vi "UHR-Fleezers Control (host) - 10.5.vi"() -> ()   [LabVIEW 2011] (continued)
                          n1375 = local read "BD 2 Frequency 3 (MHz)"() -> (w2101:dbl)
                          n1376 = local write "Trap Delta (MHz)"(w2098) -> ()
                          n1377 = call "set RF board frequency - interlace.vi"("Board 2 Frequency Limits"=w2099, "Board 1 Frequency Limits"=w2100, "FPGA VI Reference In"=w2107, "Board 2 Frequency 3 (MHz)"=w2101, "Board 1 Frequency 3 (MHz)"=w2106, "Board 2 Frequency 2 (MHz)"=w2102, "Board 2 Frequency 1 (MHz)"=w2103, "Board 1 Frequency 2 (MHz)"=w2104, "Board 1 Frequency 1  (MHz)"=w2105) -> ()  [unwired: 1 in, 2 out]
                          n1378 = local write "BD 2 Frequency 1 (MHz)"(w2103) -> ()
                          n1379 = local write "BD 1 Frequency 1 (MHz)"(w2105) -> ()
                        }
                      }
                    }
                    frame True {
                    }
                  }
                }
                event Mouse Up {
                  n1380 = event-data() -> ("Button"=w2108:u16)  [unwired: 8 out]
                  n1381 = case shown="3" w2108 {
                    tunnel: [FALSE TRUE] -> w2109
                    frame 0, Default {
                    }
                    frame 3 {
                      n1382 = local read "Trap Delta (MHz)"() -> (w2111:dbl)
                      n1383 = property on="Initial delta (MHz)" class="DigNum (strict)"("Val(Sgnl)"=w2111) -> ()  [unwired: 2 in, 2 out]
                      n1384 = local write "Manipulating Trap"(FALSE ("Manipulating Trap")) -> ()
                    }
                  }
                }
              }
            }
          }
        }
      }
      event Mouse Move {
        n1385 = event-data() -> ()  [unwired: 6 out]
      }
    }
    n1386 = local read "Stop All"() -> (w1930:bool)
    n1387 = node-c288() -> ()  [unwired: 2 out]
  }
  n1388 = timed-loop "Oscillate Trap/AOM (fishing, debugging)" {
    tunnel: w40 -> [w2115]
    tunnel: [w2114] -> w85
    timing: w80 -> [_]
    timing-out: [_] -> w79
    stop <- w2114 stop-if-true
    n1389 = node-c288() -> ()  [unwired: 2 out]
    n1390 = event shown="[0] \"Oscillate Set 1\", \"Fish for Tether\": Value Change" {
      selector: _ -> [_ _ _]
      dyn-events: _ -> [_ _ _]
      timeout: _ -> [_ _ _]
      tunnel: w2115 -> [w2122 _ _]
      tunnel: [FALSE ("Stop All") _ w2411] -> w2114
      event "Oscillate Set 1", "Fish for Tether": Value Change {
        n1391 = event-data() -> ()  [unwired: 6 out]
        n1392 = local read "Oscillate Set 1"() -> (w2121:bool)
        n1393 = Or(x=w2121, y="Fish for Tether") -> (x .or. y?=w2119:bool)
        n1394 = case shown="True" w2119 {
          tunnel: w2122 -> [_ w2125]
          tunnel: "Fish for Tether" -> [_ w2124]
          frame False {
          }
          frame True {
            n1395 = case shown="True" w2124 {
              selector: w2124 -> [w2128 w2135]
              tunnel: [w2128 w2135] -> w2123
              frame False {
              }
              frame True {
                n1396 = local write "Scan axis 2"(TRUE) -> ()
                n1397 = local write "Tether"(FALSE ("Tether")) -> ()
                n1398 = property on="Trap Delta (MHz)" class="DigNum (strict)"("Val(Sgnl)"="Furthest Delta (MHz)") -> ()  [unwired: 2 in, 2 out]
                n1399 = local read "Sample Channel\nFlow"() -> (w2132:bool)
                n1400 = Not(x=w2132) -> (.not. x?=w2130:bool)
                n1401 = And(x=w2130, y="Flow ON during \nfishing?") -> (x .and. y?=w2129:bool)
                n1402 = Wait (ms)(milliseconds to wait=u32 500) -> ()  [unwired: 1 out]
                n1403 = case shown="True" w2129 {
                  selector: w2129 -> [_ w2138]
                  frame False {
                  }
                  frame True {
                    n1404 = property on="Sample Channel\nFlow" class="Bool (strict)"("Val(Sgnl)"=w2138) -> ()  [unwired: 2 in, 2 out]
                  }
                }
              }
            }
            n1405 = node-c288() -> (w2127:T21)  [unwired: 4 out]
            n1406 = timed-loop "Oscillate AOD" {
              timing: w2127 -> [_]
              timing-out: [_] -> w2126
              tunnel: w2125 -> [w2146]
              tunnel: w2123 -> [w2139]
              i -> [w2148]
              stop <- w2145 stop-if-true
              n1407 = node-c288() -> (w2147:i64)  [unwired: 1 out]
              n1408 = flat-sequence {
                tunnel: w2148 -> [w2175]
                tunnel: w2147 -> [w2174]
                tunnel: w2146 -> [w2153]
                tunnel: w2139 -> [w2156]
                tunnel: [w2156] -> w2144
                tunnel: [w2155] -> w2143
                tunnel: [w2152] -> w2142
                tunnel: [w2149] -> w2140
                tunnel: w2144 -> [w2211]
                tunnel: w2143 -> [w2209]
                tunnel: w2142 -> [w2208]
                tunnel: [w2207] -> w2141
                tunnel: w2140 -> [w2206]
                tunnel: [w2285] -> w2145
                tunnel: w2141 -> [w2284]
                frame #0 {
                  n1409 = Divide(x=w2174, y=i64 1000) -> (x/y=w2169:dbl)
                  n1410 = Multiply(x=w2169, y=w2175) -> (x*y=w2171:dbl)
                  n1411 = local read "BD 1 Frequency 2 (MHz)"() -> (w2154:dbl)
                  n1412 = Multiply(x="Osc. freq. (Hz)", y=6.283185307179586) -> (x*y=w2172:dbl)
                  n1413 = Multiply(x=w2172, y=w2171) -> (x*y=w2151:dbl)
                  n1414 = local read "BD 1 Frequency 1 (MHz)"() -> (w2159:dbl)
                  n1415 = case shown="True" w2156 {
                    tunnel: w2151 -> [w2181 w2186]
                    tunnel: w2159 -> [_ w2197]
                    tunnel: w2154 -> [_ w2198]
                    tunnel: [w2178 w2192] -> w2157
                    tunnel: [FALSE w2189] -> w2152
                    tunnel: [0.0 w2182] -> w2149
                    frame False {
                      n1416 = Sine(x=w2181) -> (sin(x)=w2179:dbl)
                      n1417 = Multiply(x=w2179, y="Osc. amp. (MHz)") -> (x*y=w2178:dbl)
                    }
                    frame True {
                      n1418 = Cosine(x=w2186) -> (cos(x)=w2201:dbl)
                      n1419 = Subtract(x=w2198, y=w2197) -> (x-y=w2196:dbl)
                      n1420 = Decrement(x=w2201) -> (x-1=w2200:dbl)
                      n1421 = Subtract(x=w2196, y="Closest Delta (MHz)") -> (x-y=w2193:dbl)
                      n1422 = Divide(x=w2200, y=-2.0) -> (x/y=w2194:dbl)
                      n1423 = Multiply(x=w2194, y=w2193) -> (x*y=w2192:dbl)
                      n1424 = local read "Vec Mean of T1 T2"() -> (w2188:dbl[])
                      n1425 = Greater?(x=w2188, y="Stop F (pN)") -> (0:w2190:bool[])
                      n1426 = Or Array Elements(Boolean array=w2190) -> (logical OR=w2189:bool)
                      n1427 = Divide(x=w2186, y=6.283185307179586) -> (x/y=w2185:dbl)
                      n1428 = Round Toward +Infinity(x=w2185) -> (ceil(x): smallest int >= x=w2182:dbl)
                      "Attempts" <- w2182
                      n1429 = Greater?(x=w2182, y="Attempt Limit") -> (0:w2184:bool)
                      n1430 = case shown="True" w2184 {
                        frame False {
                        }
                        frame True {
                          n1431 = local write "Fish for Tether"(FALSE ("Fish for Tether")) -> ()
                          n1432 = call <vilib>:"Beep.vi"() -> ()  [unwired: 3 in, 9 out]
                          n1433 = local read "Messages"() -> (w2203:string)
                          n1434 = call "Update messages.vi"("Message to add"="Tether fishing timeout." ("Messages"), "Old message string"=w2203) -> ("New message string"=→"Messages":string)
                        }
                      }
                    }
                  }
                  n1435 = local read "BD 2 Frequency 1 (MHz)"() -> (w2158:dbl)
                  n1436 = Select(t=w2159, s="Scan axis 2", f=w2158) -> (s? t:f=w2162:dbl)
                  n1437 = Add(x=w2157, y=w2162) -> (x+y=w2155:dbl)
                  n1438 = Select(t=w2155, s="Scan axis 2", f=w2159) -> (s? t:f=w2165:dbl)
                  n1439 = Select(t=w2158, s="Scan axis 2", f=w2155) -> (s? t:f=w2164:dbl)
                  n1440 = local read "Y RF Frequency Limits (MHz)"() -> (w2160:T16)
                  n1441 = local read "X RF Frequency Limits (MHz)"() -> (w2161:T16)
                  n1442 = local read "BD 1 Frequency 3 (MHz)"() -> (w2168:dbl)
                  n1443 = local read "BD 2 Frequency 2 (MHz)"() -> (w2167:dbl)
                  n1444 = local read "BD 2 Frequency 3 (MHz)"() -> (w2166:dbl)
                  n1445 = call "set RF board frequency - interlace.vi"("Board 2 Frequency Limits"=w2160, "Board 1 Frequency Limits"=w2161, "FPGA VI Reference In"=w2153, "Board 2 Frequency 3 (MHz)"=w2166, "Board 1 Frequency 3 (MHz)"=w2168, "Board 2 Frequency 2 (MHz)"=w2167, "Board 2 Frequency 1 (MHz)"=w2164, "Board 1 Frequency 2 (MHz)"=w2154, "Board 1 Frequency 1  (MHz)"=w2165) -> ()  [unwired: 1 in, 2 out]
                }
                frame #1 {
                  n1446 = And(x=w2211, y=w2208) -> (x .and. y?=w2210:bool)
                  n1447 = case "Only if were fishing and now formed tether" shown="True" w2210 {
                    tunnel: w2209 -> [w2213 w2230]
                    tunnel: [w2212 w2229] -> w2207
                    tunnel: w2206 -> [_ w2225]
                    frame False {
                      n1448 = local read "Fish for Tether"() -> (w2212:bool)
                      n1449 = case shown="False" w2212 {
                        tunnel: w2213 -> [w2214 _]
                        frame False {
                          n1450 = property on="BD 1 Frequency 1 (MHz)" class="DigNum (strict)"("Val(Sgnl)"=w2214) -> ()  [unwired: 2 in, 2 out]
                        }
                        frame True {
                        }
                      }
                    }
                    frame True {
                      w2229 = FALSE ("Fish for Tether")
                      n1451 = call <vilib>:"Beep.vi"() -> ()  [unwired: 3 in, 9 out]
                      n1452 = Number To Decimal String(number=w2225, width (-)=i16 1) -> (decimal integer string=w2223:string)
                      n1453 = Concatenate Strings("Formed tether in ", w2223, " attempt(s)." ("string")) -> (w2220:string)
                      n1454 = local read "Messages"() -> (w2227:string)
                      n1455 = local write "Fish for Tether"(w2229) -> ()
                      n1456 = call "Update messages.vi"("Message to add"=w2220, "Old message string"=w2227) -> ("New message string"=w2226:string)
                      n1457 = local write "Messages"(w2226) -> ()
                      n1458 = Get Date/Time In Seconds() -> (seconds since 1Jan1904=→"Time tether formed":timestamp)
                      n1459 = local read "Sample Channel\nFlow"() -> (w2218:bool)
                      n1460 = local read "Flow ON during \nfishing?"() -> (w2217:bool)
                      n1461 = And(x=w2218, y=w2217) -> (x .and. y?=w2216:bool)
                      n1462 = case shown="True" w2216 {
                        tunnel: [_ w2232] -> w2215
                        frame False {
                        }
                        frame True {
                          n1463 = property on="Sample Channel\nFlow" class="Bool (strict)"("Val(Sgnl)"=FALSE ("Value (Signaling)")) -> (error out=w2232:errorcluster)  [unwired: 2 in, 1 out]
                        }
                      }
                      n1464 = case shown="\"2\", \"3\", \"4\", \"5\", \"6\"" "Then..." {
                        selector: "Then..." -> [_ w2235]
                        tunnel: w2230 -> [w2234 _]
                        tunnel: w2215 -> [_ _]
                        frame "1", Default {
                          n1465 = property on="BD 1 Frequency 1 (MHz)" class="DigNum (strict)"("Val(Sgnl)"=w2234) -> ()  [unwired: 2 in, 2 out]
                        }
                        frame "2", "3", "4", "5", "6" {
                          n1466 = flat-sequence {
                            tunnel: w2235 -> [w2237]
                            frame #0 {
                              n1467 = property on="Trap Delta (MHz)" class="DigNum (strict)"("Val(Sgnl)"="Move to Delta 1 (MHz)") -> ()  [unwired: 2 in, 2 out]
                            }
                            frame #1 {
                              n1468 = case shown="\"5\", \"6\"" w2237 {
                                selector: w2237 -> [w2240 w2250 _]
                                frame "3", "4" {
                                n1469 = flat-sequence {
                                tunnel: w2240 -> [w2241]
                                tunnel: [w2241] -> w2238
                                tunnel: [w2243] -> w2239
                                tunnel: w2238 -> [w2243]
                                tunnel: w2239 -> [w2247]
                                frame #0 {
                                n1470 = property on="Green Laser ON/Interlacing" class="Bool (strict)"("Val(Sgnl)"=TRUE ("Value (Signaling)")) -> ()  [unwired: 2 in, 2 out]
                                }
                                frame #1 {
                                n1471 = Multiply(x="Wait Before Save (s)", y=u32 1000 ("x")) -> (x*y=w2245:u32)
                                n1472 = Wait (ms)(milliseconds to wait=w2245) -> ()  [unwired: 1 out]
                                }
                                frame #2 {
                                n1473 = property on="Start Saving" class="Bool (strict)"("Value"=TRUE ("Start Saving")) -> ()  [unwired: 2 in, 2 out]
                                n1474 = case shown="\"4\"" w2247 {
                                frame Default {
                                }
                                frame "4" {
                                n1475 = property on="Fl. Triggered..." class="Bool (strict)"("Val(Sgnl)"=TRUE ("Value (Signaling)")) -> ()  [unwired: 2 in, 2 out]
                                }
                                }
                                }
                                }
                                }
                                frame "5", "6" {
                                n1476 = stacked-sequence {
                                tunnel: w2250 -> [_ _ _ _ _ _ w2262]
                                frame #0 {
                                n1477 = Replace Array Subset(array=u32[] [0] ("Index Values"), new element="Raster Set Upon Tether", index=0) -> (w2251:u32[])
                                n1478 = property on="Saved AOD Raster Scan Parameter Sets" class="Arr (strict)"("Index Values"=w2251) -> ()  [unwired: 2 in, 2 out]
                                }
                                frame #1 {
                                n1479 = Wait (ms)(milliseconds to wait=u32 500) -> ()  [unwired: 1 out]
                                }
                                frame #2 {
                                n1480 = property on="Load parameters" class="Bool (strict)"("Val(Sgnl)"=TRUE ("Value (Signaling)")) -> ()  [unwired: 2 in, 2 out]
                                n1481 = case shown="True" "Green ON During Raster" {
                                frame False {
                                }
                                frame True {
                                n1482 = property on="Green Laser ON/Interlacing" class="Bool (strict)"("Val(Sgnl)"=TRUE ("Value (Signaling)")) -> ()  [unwired: 2 in, 2 out]
                                }
                                }
                                }
                                frame #3 {
                                n1483 = Wait (ms)(milliseconds to wait=u32 500) -> ()  [unwired: 1 out]
                                }
                                frame #4 {
                                n1484 = property on="Trap Raster Scan" class="Bool (strict)"("Val(Sgnl)"=TRUE ("Value (Signaling)")) -> ()  [unwired: 2 in, 2 out]
                                }
                                frame #5 {
                                n1485 = Wait (ms)(milliseconds to wait=u32 2000) -> ()  [unwired: 1 out]
                                }
                                frame #6 {
                                n1486 = flat-sequence {
                                tunnel: w2262 -> [w2269]
                                frame #0 {
                                n1487 = while {
                                stop <- w2265 stop-if-true
                                n1488 = local read "Raster Scanning..."() -> (w2264:bool)
                                n1489 = local read "Saving..."() -> (w2267:bool)
                                n1490 = Wait (ms)(milliseconds to wait=u32 100) -> ()  [unwired: 1 out]
                                n1491 = Not(x=w2267) -> (.not. x?=w2266:bool)
                                n1492 = Not(x=w2264) -> (.not. x?=w2263:bool)
                                n1493 = And(x=w2266, y=w2263) -> (x .and. y?=w2265:bool)
                                }
                                }
                                frame #1 {
                                n1494 = local read "Tether"() -> (w2270:bool)
                                n1495 = case shown="False" w2270 {
                                tunnel: w2269 -> [_ w2272]
                                frame False {
                                n1496 = property on="Fish for Tether" class="Bool (strict)"("Val(Sgnl)"="Fish again after \nraster break?") -> ()  [unwired: 2 in, 2 out]
                                }
                                frame True {
                                n1497 = stacked-sequence {
                                tunnel: w2272 -> [_ w2274 _ _]
                                frame #0 {
                                n1498 = property on="Trap Delta (MHz)" class="DigNum (strict)"("Val(Sgnl)"="Move to Delta 2 (MHz)") -> ()  [unwired: 2 in, 2 out]
                                }
                                frame #1 {
                                n1499 = flat-sequence {
                                tunnel: w2274 -> [w2276]
                                frame #0 {
                                n1500 = Wait (ms)(milliseconds to wait=u32 500) -> ()  [unwired: 1 out]
                                }
                                frame #1 {
                                n1501 = case shown="\"6\"" w2276 {
                                frame Default {
                                }
                                frame "6" {
                                n1502 = property on="Green Laser ON/Interlacing" class="Bool (strict)"("Val(Sgnl)"=TRUE ("Green Laser ON/Interlacing")) -> ()  [unwired: 2 in, 2 out]
                                }
                                }
                                }
                                frame #2 {
                                n1503 = Wait (ms)(milliseconds to wait=u32 500) -> ()  [unwired: 1 out]
                                }
                                frame #3 {
                                n1504 = local write "Start Saving"("Save at end (5, 6)") -> ()
                                }
                                }
                                }
                                frame #2 {
                                n1505 = local read "Bead Sep. Int. Time (s)"() -> (w2282:dbl)
                                n1506 = Multiply(x=w2282, y=1000.0) -> (x*y=w2281:dbl)
                                n1507 = Wait (ms)(milliseconds to wait=w2281) -> ()  [unwired: 1 out]
                                }
                                frame #3 {
                                n1508 = property on="Remove Offset" class="Bool (strict)"("Val(Sgnl)"=TRUE ("Value (Signaling)")) -> ()  [unwired: 2 in, 2 out]
                                }
                                }
                                }
                                }
                                }
                                }
                                }
                                }
                                }
                                frame "2", Default {
                                }
                              }
                            }
                          }
                        }
                      }
                      "Tether" <- "Tether Alarm?"
                    }
                  }
                }
                frame #2 {
                  n1509 = local read "Oscillate Set 1"() -> (w2289:bool)
                  n1510 = local read "Stop All"() -> (w2287:bool)
                  n1511 = Or(x=w2289, y=w2284) -> (x .or. y?=w2286:bool)
                  n1512 = Not(x=w2286) -> (.not. x?=w2288:bool)
                  n1513 = Compound Arithmetic op=OR(w2287, w2288) -> (w2285:bool)
                }
              }
              n1514 = node-c288() -> ()  [unwired: 2 out]
            }
            n1515 = node-c288(w2126) -> ()  [unwired: 1 out]
          }
        }
      }
      event "Fl. Triggered...": Value Change {
        n1516 = event-data() -> ()  [unwired: 7 out]
        n1517 = case shown="True" "Fl. Triggered..." {
          frame False {
          }
          frame True {
            n1518 = node-c288() -> (w2299:T21)  [unwired: 4 out]
            n1519 = timed-loop {
              timing: w2299 -> [_]
              timing-out: [_] -> w2298
              tunnel: "Action" -> [w2303]
              shift-right: [w2300] -> _
              shift-left: u8 255 -> [w2302]
              stop <- w2304 stop-if-true
              n1520 = node-c288() -> ()  [unwired: 2 out]
              n1521 = flat-sequence {
                tunnel: w2303 -> [w2316]
                tunnel: w2302 -> [w2313]
                tunnel: [w2312] -> w2301
                tunnel: [w2402] -> w2304
                tunnel: w2301 -> [w2401]
                tunnel: [w2401] -> w2300
                frame #0 {
                  n1522 = local read "Delta Fl. 2"() -> (w2307:dbl)
                  n1523 = local read "Delta Fl. 1"() -> (w2308:dbl)
                  n1524 = Select(t=w2308, s="APD to Watch", f=w2307) -> (s? t:f=w2306:dbl)
                  n1525 = Multiply(x="Fl. Delta Thresh. (kHz)", y=1000.0) -> (x*y=w2315:dbl)
                  n1526 = Greater?(x=w2306, y=w2315) -> (0:w2310:bool)
                  n1527 = Or(x="Force Yank", y=w2310) -> (x .or. y?=w2311:bool)
                  n1528 = case shown="True" w2311 {
                    tunnel: w2316 -> [_ w2326]
                    tunnel: w2313 -> [w2318 w2322]
                    tunnel: [w2318 w2319] -> w2312
                    frame False {
                    }
                    frame True {
                      n1529 = flat-sequence {
                        tunnel: w2323 -> [w2332]
                        tunnel: [w2332] -> w2327
                        tunnel: w2326 -> [w2331]
                        tunnel: [w2331] -> w2325
                        tunnel: [w2330] -> w2324
                        tunnel: w2322 -> [w2329]
                        tunnel: [w2328] -> w2321
                        tunnel: w2327 -> [w2357]
                        tunnel: w2325 -> [w2356]
                        tunnel: w2324 -> [w2355]
                        tunnel: w2321 -> [w2354]
                        tunnel: [w2354] -> w2320
                        tunnel: w2320 -> [w2399]
                        tunnel: [w2399] -> w2319
                        frame #0 {
                          n1530 = call <vilib>:"Beep.vi"() -> ()  [unwired: 3 in, 9 out]
                          n1531 = local write "Waiting"(FALSE ("Waiting")) -> ()
                          n1532 = Increment(x=w2329) -> (x+1=w2328:u8)
                          n1533 = case shown="\"Yank\"" w2331 {
                            tunnel: w2328 -> [_ _ w2338]
                            frame "Image" {
                              n1534 = property on="Confocal Image" class="Bool (strict)"("Val(Sgnl)"=TRUE ("Value (Signaling)")) -> ()  [unwired: 2 in, 2 out]
                            }
                            frame "Alarm", Default {
                            }
                            frame "Yank" {
                              n1535 = flat-sequence {
                                tunnel: w2338 -> [w2341]
                                tunnel: [w2340] -> w2337
                                tunnel: ["N Array El"] -> w2336
                                tunnel: w2337 -> [w2351]
                                tunnel: w2336 -> [w2347]
                                frame #0 {
                                n1536 = Multiply(x="Yank Delay (s)", y=1000.0) -> (x*y=w2344:dbl)
                                n1537 = Quotient & Remainder(x=w2341, y="N Array El") -> (x-y*floor(x/y)=w2340:u8)  [unwired: 1 out]
                                n1538 = Wait (ms)(milliseconds to wait=w2344) -> ()  [unwired: 1 out]
                                }
                                frame #1 {
                                n1539 = Random Number (0-1)() -> (number: 0 to 1=w2348:dbl)
                                n1540 = Multiply(x=w2347, y=w2348) -> (x*y=w2346:dbl)
                                n1541 = Round Toward -Infinity(1:w2346) -> (0:w2345:dbl)
                                n1542 = Select(t=w2345, s="Random Choice", f=w2351) -> (s? t:f=w2349:dbl)
                                n1543 = Index Array(array="Yank to Delta Array (MHz)", index=w2349) -> (element=w2352:dbl)
                                n1544 = property on="Trap Delta (MHz)" class="DigNum (strict)"("Val(Sgnl)"=w2352) -> ()  [unwired: 2 in, 2 out]
                                }
                              }
                            }
                          }
                          n1545 = local read "Time (s)"() -> (w2330:dbl)
                          "Fl. High" <- TRUE ("Yanking")
                        }
                        frame #1 {
                          n1546 = node-c288() -> (w2359:T21)  [unwired: 4 out]
                          n1547 = timed-loop {
                            timing: w2359 -> [_]
                            timing-out: [_] -> w2358
                            tunnel: w2357 -> [w2375]
                            tunnel: w2356 -> [w2373]
                            tunnel: w2355 -> [w2372]
                            stop <- w2374 stop-if-true
                            n1548 = node-c288() -> ()  [unwired: 2 out]
                            n1549 = local read "Fl. Delta Thresh. (kHz)"() -> (w2367:dbl)
                            n1550 = local read "Fl. Triggered..."() -> (w2376:bool)
                            n1551 = local read "Delta Fl. 1"() -> (w2363:dbl)
                            n1552 = local read "Delta Fl. 2"() -> (w2361:dbl)
                            n1553 = local read "Stop All"() -> (w2370:bool)
                            n1554 = local read "APD to Watch"() -> (w2362:bool)
                            n1555 = Select(t=w2363, s=w2362, f=w2361) -> (s? t:f=w2360:dbl)
                            n1556 = Not(x=w2376) -> (.not. x?=w2371:bool)
                            n1557 = Multiply(x=w2367, y=1000.0) -> (x*y=w2366:dbl)
                            n1558 = Negate(x=w2366) -> (-x=w2365:dbl)
                            n1559 = Less?(x=w2360, y=w2365) -> (x < y?=w2369:bool)
                            n1560 = Compound Arithmetic op=OR(w2369, w2370, w2371, "Force Reset") -> (w2374:bool)
                            n1561 = case shown="True" w2374 {
                              tunnel: w2375 -> [_ w2387]
                              tunnel: w2373 -> [_ w2386]
                              tunnel: w2372 -> [_ w2384]
                              frame False {
                              }
                              frame True {
                                n1562 = case shown="\"Yank\"" w2386 {
                                tunnel: w2387 -> [_ w2388]
                                frame "Image", Default {
                                }
                                frame "Yank" {
                                n1563 = flat-sequence {
                                tunnel: [w2393] -> w2389
                                tunnel: w2388 -> [w2393]
                                tunnel: w2389 -> [w2394]
                                frame #0 {
                                n1564 = local read "Yank Delay (s)"() -> (w2392:dbl)
                                n1565 = Multiply(x=w2392, y=1000.0) -> (x*y=w2390:dbl)
                                n1566 = Wait (ms)(milliseconds to wait=w2390) -> ()  [unwired: 1 out]
                                }
                                frame #1 {
                                n1567 = property on="Trap Delta (MHz)" class="DigNum (strict)"("Val(Sgnl)"=w2394) -> ()  [unwired: 2 in, 2 out]
                                }
                                }
                                }
                                }
                                n1568 = local read "Time (s)"() -> (w2385:dbl)
                                n1569 = Subtract(x=w2385, y=w2384) -> (x-y=w2381:dbl)
                                "Duration (s)" <- w2381
                                n1570 = Number To Decimal String(number=w2381, width (-)=i16 0) -> (decimal integer string=w2379:string)
                                n1571 = Concatenate Strings(w2379, " s fluorescence event." ("string")) -> (w2377:string)
                                n1572 = local read "Messages"() -> (w2383:string)
                                n1573 = call "Update messages.vi"("Message to add"=w2377, "Old message string"=w2383) -> ("New message string"=w2382:string)
                                n1574 = call <vilib>:"Beep.vi"() -> ()  [unwired: 3 in, 9 out]
                                n1575 = local write "Messages"(w2382) -> ()
                              }
                            }
                            n1576 = node-c288() -> ()  [unwired: 2 out]
                          }
                          n1577 = node-c288(w2358) -> ()  [unwired: 1 out]
                        }
                        frame #2 {
                          n1578 = local write "Fl. High"(FALSE ("Yanking")) -> ()
                        }
                      }
                      n1579 = local read "Trap Delta (MHz)"() -> (w2323:dbl)
                    }
                  }
                }
                frame #1 {
                  n1580 = local read "Stop All"() -> (w2405:bool)
                  n1581 = local read "Fl. Triggered..."() -> (w2403:bool)
                  n1582 = Not(x=w2403) -> (.not. x?=w2404:bool)
                  n1583 = Or(x=w2404, y=w2405) -> (x .or. y?=w2402:bool)
                  n1584 = Not(x=w2402) -> (.not. x?=→"Waiting":bool)
                }
              }
              n1585 = node-c288() -> ()  [unwired: 2 out]
            }
            n1586 = node-c288(w2298) -> ()  [unwired: 1 out]
          }
        }
      }
      event "Stop All": Value Change {
        n1587 = event-data() -> ()  [unwired: 7 out]
        n1588 = local read "Stop All"() -> (w2411:bool)
      }
    }
    n1589 = node-c288() -> ()  [unwired: 2 out]
  }
  n1590 = flat-sequence "Video" {
    tunnel: [w2420] -> w70
    tunnel: w70 -> [w2461]
    frame #0 {
      n1591 = while {
        stop <- w2413 continue-if-true
        n1592 = call "Close Video Capture.vi"() -> ("error code OUT"=w2415:i32)
        n1593 = Equal?(x=w2415, y=0) -> (x = y?=w2413:bool)
      }
      n1594 = local write "Stop All"(FALSE ("Stop All")) -> ()
    }
    frame #1 {
      n1595 = call "DMR_Init.vi"() -> ()  [unwired: 3 out]
    }
    frame #2 {
      # "Setting the destination format to Mono8 makes sure that the image can be displayed in the intensity plot."
      n1596 = call "DMR_GetDevice.vi"("search string IN"="DE019116701") -> ("device handle OUT"=w2438:i32)  [unwired: 4 in, 2 out]
      n1597 = call "DMR_OpenDevice.vi"("device handle IN"=w2438) -> ("driver handle OUT"=w2421:i32)  [unwired: 4 out]
      n1598 = call "DMR_FindList.vi"("flags IN"=u32 0 ("flags"), "list name IN"="" ("String"), "list type IN"=T31."camera descriptions", "driver handle IN"=w2421) -> ("list handle OUT"=w2424:i32)  [unwired: 2 out]
      n1599 = call "DMR_FindList.vi"("flags IN"=u32 0 ("flags"), "list name IN"="Base", "list type IN"=T31."setting", "driver handle IN"=w2421) -> ("list handle OUT"=w2422:i32)  [unwired: 2 out]
      n1600 = call "OBJ_GetHandle.vi"("object name IN"="VideoStandard", "list handle IN"=w2424) -> ("object handle OUT"=w2418:i32)  [unwired: 3 out]
      n1601 = call "OBJ_GetHandle.vi"("object name IN"="PixelFormat", "list handle IN"=w2422) -> ("object handle OUT"=w2432:i32)  [unwired: 3 out]
      n1602 = call "OBJ_SetS.vi"("value index IN"=0, "value IN"="NTSC M", "object handle IN"=w2418) -> ()  [unwired: 2 out]
      n1603 = call "OBJ_SetS.vi"("value index IN"=0, "value IN"="Mono8" ("value"), "object handle IN"=w2432) -> ()  [unwired: 2 out]
      n1604 = call "OBJ_GetHandle.vi"("object name IN"="VideoChannel", "list handle IN"=w2422) -> ("object handle OUT"=w2428:i32)  [unwired: 3 out]
      n1605 = while {
        tunnel: [w2443] -> w2420
        tunnel: w2421 -> [w2440]
        stop <- w2441 continue-if-true
        n1606 = call "DMR_ImageRequestSingle.vi"("request control IN"=0, "driver handle IN"=w2440) -> ("error code OUT"=w2442:i32, "driver handle OUT"=w2443:i32)  [unwired: 2 out]
        n1607 = Equal To 0?(x=w2442) -> (x = 0?=w2441:bool)
      }
      n1608 = call "OBJ_SetI.vi"("value index IN"=0, "value IN"=3 ("Video channel"), "object handle IN"=w2428) -> ()  [unwired: 2 out]
    }
    frame #3 {
      w2449 = T17 0 items=["Grayscale (U8)", "Grayscale (I16)", "Grayscale (SGL)", "Complex (CSG)", "RGB (U32)", "HSL (U32)", "RGB (U64)"] ("Image Type")
      w2457 = T17 0 items=["Grayscale (U8)", "Grayscale (I16)", "Grayscale (SGL)", "Complex (CSG)", "RGB (U32)", "HSL (U32)", "RGB (U64)"] ("Image Type")
      n1609 = for "Create Greyscale map" {
        N: 256 -> [_]
        tunnel: [w2463] -> w2446 mode=indexing
        workers-P: _ -> [_]
        i -> [w2466]
        n1610 = To Unsigned Byte Integer(number=w2466) -> (unsigned 8bit integer=w2462:u8)
        n1611 = Join Numbers(hi=w2462, lo=w2462) -> ((hi.lo)=w2465:u16)
        n1612 = Join Numbers(hi=w2462, lo=w2462) -> ((hi.lo)=w2464:u16)
        n1613 = Join Numbers(hi=w2465, lo=w2464) -> ((hi.lo)=w2463:u32)
      }
      n1614 = call "IMAQ Create"("Image Name"="Scaled video", "Image Type"=w2449) -> ("New Image"=w2448:T3)  [unwired: 2 in, 2 out]
      n1615 = call "IMAQ Create"("Image Name"="Main video", "Image Type"=w2457) -> ("New Image"=w2458:T3)  [unwired: 2 in, 2 out]
      n1616 = node-c288(0 ("Processor")) -> (w2456:T21)  [unwired: 3 out]
      n1617 = Initialize Array(u32 0 ("Window Number (0...15)"), 480 ("dimension size"), 640 ("dimension size")) -> (w2451:u32[][])
      n1618 = timed-loop {
        tunnel: w2461 -> [w2483]
        tunnel: [w2482] -> w2460
        tunnel: w2458 -> [w2481]
        timing: w2456 -> [_]
        timing-out: [_] -> w2455
        tunnel: w2451 -> [w2470]
        tunnel: w2448 -> [w2468]
        tunnel: w2446 -> [w2467]
        stop <- w2469 stop-if-true
        # "This block performs the \nactual image capture."
        n1619 = node-c288() -> ()  [unwired: 2 out]
        n1620 = local read "Stop All"() -> (w2469:bool)
        n1621 = Reciprocal(x="Video Capture Rate (Hz)") -> (1/x=w2473:dbl)
        n1622 = Multiply(x=w2473, y=1000.0) -> (x*y=w2471:dbl)
        n1623 = call "DMR_ImageRequestWaitFor.vi"("queue number IN"=0, "timeout(ms) IN"=500, "driver handle IN"=w2483) -> ("error code OUT"=w2487:i32, "request number OUT"=w2484:i32, "driver handle OUT"=w2485:i32)
        n1624 = feedback #1(T32 refnum ("Avi Refnum")) -> (w2475:T32)
        n1625 = case shown="True" "New Video File" {
          tunnel: [T32 refnum ("Avi Refnum") w2504] -> w2477
          tunnel: [FALSE TRUE] -> w2478
          tunnel: w2475 -> [_ w2500]
          frame False {
          }
          frame True {
            n1626 = call "Create new save file.vi"("Ext"=".avi" ("string"), "Index In"="Video Index") -> ("Path Out"=w2496:path, "Index Out"=w2497:dbl)  [unwired: 1 in]
            "Path Out" <- w2496
            n1627 = Not Equal?(x=w2500, y=T32 refnum ("Avi Refnum")) -> (x != y?=w2501:bool)
            n1628 = Increment(x=w2497) -> (x+1=w2506:dbl)
            n1629 = case shown="True" w2501 {
              tunnel: w2500 -> [_ w2507]
              frame False {
              }
              frame True {
                n1630 = call "IMAQ AVI Close"("Avi Refnum"=w2507) -> ()  [unwired: 1 in, 10 out]
              }
            }
            n1631 = local write "Video Index"(w2506) -> ()
            n1632 = call "IMAQ AVI Create"("Frames Per Second"=u32 30, "AVI Path"=w2496) -> ("Avi Refnum"=w2504:T32)  [unwired: 5 in, 4 out]
          }
        }
        n1633 = Equal To 0?(x=w2487) -> (x = 0?=w2486:bool)
        n1634 = Select(t=w2477, s=w2478, f=w2475) -> (s? t:f=w2476:T32)
        n1635 = feedback-in #1(w2476) -> ()
        n1636 = case shown="True" w2486 {
          tunnel: w2485 -> [w2508 w2533]
          tunnel: w2484 -> [_ w2532]
          tunnel: [w2508 w2529] -> w2482
          tunnel: w2481 -> [_ w2513]
          tunnel: w2470 -> [_ w2517]
          tunnel: w2476 -> [_ w2515]
          tunnel: w2468 -> [_ w2510]
          tunnel: w2467 -> [_ w2509]
          frame False {
          }
          frame True {
            w2523 = u32 0 ("X-offset IN")
            n1637 = call "DMR_GetImageRequestBufferData.vi"("driver handle IN"=w2533, "request number IN"=w2532) -> ("width OUT"=w2522:i32, "height OUT"=w2521:i32, "driver handle OUT"=w2528:i32, "request number OUT"=w2527:i32, "bytes per pixel OUT"=w2524:i32)  [unwired: 13 out]
            n1638 = call "DMR_GetImageRequestBufferImageData.vi"("driver handle IN"=w2528, "request number IN"=w2527, "bytes per pixel IN"=w2524, "X-offset IN"=w2523, "Y-offset IN"=w2523, "height IN"=w2521, "width IN"=w2522) -> ("driver handle OUT"=w2526:u32, "request number OUT"=w2525:u32, "image OUT"=w2518:u32[][])  [unwired: 10 out]
            n1639 = call "DMR_ImageRequestUnlock.vi"("request number IN"=w2525, "driver handle IN"=w2526) -> ("driver handle OUT"=w2531:i32)  [unwired: 1 in, 2 out]
            n1640 = case shown="True" "Averaging" {
              tunnel: w2518 -> [w2569 w2574]
              tunnel: [w2569 w2573] -> w2514
              tunnel: w2517 -> [_ w2571]
              frame False {
              }
              frame True {
                (unwired) 1
                w2579 = 1
                n1641 = feedback #2(w2571) -> (w2570:u32[][])
                n1642 = Add(x=w2574, y=w2570) -> (x+y=w2575:u32[][])
                n1643 = Select(t=w2571, s="Reset Averaging", f=w2575) -> (s? t:f=w2577:u32[][])
                n1644 = feedback-in #2(w2577) -> ()
                n1645 = feedback #3(w2579) -> (w2572:i32)
                n1646 = Divide(x=w2575, y=w2572) -> (x/y=w2576:dbl[][])
                n1647 = Increment(x=w2572) -> (x+1=w2580:i32)
                n1648 = To Unsigned Long Integer(number=w2576) -> (unsigned 32bit integer=w2573:u32[][])
                n1649 = Select(t=w2579, s="Reset Averaging", f=w2580) -> (s? t:f=w2578:i32)
                n1650 = feedback-in #3(w2578) -> ()
              }
            }
            n1651 = call "DMR_ImageRequestSingle.vi"("request control IN"=0, "driver handle IN"=w2531) -> ("driver handle OUT"=w2529:i32)  [unwired: 3 out]
            n1652 = disable-structure shown="Disabled" {
              disable-tunnel: w2514 -> [w2546 _]
              disable-tunnel: w2510 -> [w2545 _]
              frame Disabled {
                n1653 = To Double Precision Float(number=w2546) -> (double precision float=w2544:dbl[][])
                n1654 = In Range and Coerce(upper limit="Intensity Upper", x=w2544, lower limit="Intensity Lower") -> (coerced(x)=w2543:dbl[][])  [unwired: 1 out]
                n1655 = Subtract(x="Intensity Upper", y="Intensity Lower") -> (x-y=w2540:dbl)
                n1656 = Subtract(x=w2543, y="Intensity Lower") -> (x-y=w2541:dbl[][])
                n1657 = Divide(x=w2541, y=w2540) -> (x/y=w2542:dbl[][])
                n1658 = Multiply(x=255.0, y=w2542) -> (x*y=w2538:dbl[][])
                n1659 = To Unsigned Byte Integer(number=w2538) -> (unsigned 8bit integer=w2547:u8[][])
                n1660 = call "IMAQ ArrayToImage"("Image Pixels (U8)"=w2547, "Image"=w2545) -> ("Image Out"=w2534:T3)  [unwired: 4 in, 5 out]
                n1661 = First Call?() -> (First Call?: T/F=w2535:bool)
                n1662 = case shown="True" w2535 {
                  tunnel: w2534 -> [w2548 w2559]
                  frame False {
                    n1663 = flat-sequence {
                      tunnel: w2548 -> [w2554]
                      frame #0 {
                        w2551 = FALSE ("Get/Set Status? (Set)")
                        w2550 = 0 ("Window Number (0...15)")
                        n1664 = call "IMAQ WindSize"("Get/Set Status? (Set)"=w2551, "Window Number"=w2550) -> ("Width & Height out"=→"Window Size":cluster{"Width":i32, "Height":i32})  [unwired: 4 in, 2 out]
                        n1665 = call "IMAQ WindMove"("Window Number (0...15)"=w2550, "Get/Set Status? (Set)"=w2551) -> ("Coordinates (screen)"=→"Window Position":cluster{"X Position":i32, "Y Position":i32})  [unwired: 3 in, 1 out]
                        n1666 = call "IMAQ WindDraw"("Resize to Image Size? (Y)"=FALSE, "Window Number (0...15)"=w2550, "Image"=w2554) -> ()  [unwired: 7 in, 2 out]
                      }
                      frame #1 {
                        n1667 = call "IMAQ WindZoom 2"("Center Point"="Center Point", "Zoom to Fit? (False)"=FALSE, "Zoom Factor"="Zoom Factor") -> ()  [unwired: 5 in, 4 out]
                      }
                    }
                  }
                  frame True {
                    n1668 = flat-sequence {
                      tunnel: w2559 -> [w2562]
                      tunnel: [w2560] -> w2558
                      tunnel: w2558 -> [w2564]
                      frame #0 {
                        w2561 = TRUE ("Resize to Image Size? (Y)")
                        w2560 = 0 ("Window Number (0...15)")
                        n1669 = call "IMAQ WindNonTearing"("Window Number"=w2560, "NonTearing? (True)"=w2561) -> ()  [unwired: 8 in, 2 out]
                        n1670 = call "IMAQ WindDraw"("Resize to Image Size? (Y)"=w2561, "Window Number (0...15)"=w2560, "Image"=w2562) -> ()  [unwired: 7 in, 2 out]
                      }
                      frame #1 {
                        n1671 = call "IMAQ WindSize"("Scrollbars? (N)"=FALSE, "Width & Height"="Initial Window Size", "Window Number"=w2564) -> ()  [unwired: 3 in, 3 out]
                        n1672 = call "IMAQ WindMove"("Window Number (0...15)"=w2564, "Coordinates (screen)"="Initial Window Position") -> ()  [unwired: 3 in, 2 out]
                      }
                    }
                  }
                }
              }
              frame Enabled {
              }
            }
            n1673 = To Unsigned Byte Integer(number=w2514) -> (unsigned 8bit integer=w2512:u8[][])
            n1674 = call "IMAQ ArrayToImage"("Image Pixels (U8)"=w2512, "Image"=w2513) -> ("Image Out"=w2511:T3)  [unwired: 4 in, 5 out]
            "Primary Video Display" <- w2511
            n1675 = case shown="True" "Save Video" {
              tunnel: w2515 -> [_ w2568]
              tunnel: w2511 -> [_ w2567]
              frame False {
              }
              frame True {
                n1676 = call "IMAQ AVI Write Frame"("Image"=w2567, "Avi Refnum"=w2568) -> ()  [unwired: 2 in, 8 out]
              }
            }
            n1677 = case shown="True" "Save Image" {
              tunnel: w2512 -> [_ w2583]
              tunnel: w2509 -> [_ w2582]
              frame False {
              }
              frame True {
                n1678 = call <vilib>:"Flatten Pixmap.vi"("colors"=w2582, "8-bit pixmap"=w2583) -> ("image data"=w2589:T33)  [unwired: 4 in, 5 out]
                n1679 = call "Create new save file.vi"("Insert"="video_frame_" ("string"), "Ext"=".bmp" ("string"), "Index In"="Image Index") -> ("Path Out"=w2585:path, "Index Out"=w2590:dbl)
                n1680 = Increment(x=w2590) -> (x+1=w2584:dbl)
                n1681 = local write "Image Index"(w2584) -> ()
                n1682 = call <vilib>:"Write BMP File.vi"("image data"=w2589, "path to BMP file"=w2585) -> ()  [unwired: 1 in, 9 out]
              }
            }
          }
        }
        n1683 = node-c288(w2471) -> ()  [unwired: 1 out]
      }
      n1684 = node-c288(w2455) -> ()  [unwired: 1 out]
      n1685 = call "DMR_CloseDevice.vi"("driver handle IN"=w2460) -> ()  [unwired: 1 in, 4 out]
    }
    frame #4 {
      n1686 = call "DMR_Close.vi"() -> ()  [unwired: 1 out]
    }
  }
  n1687 = node-c288(i64 1 ("Period"), 1 ("Processor")) -> (w165:T21)  [unwired: 2 out]
  n1688 = timed-loop "Acquire Data" {
    tunnel: w40 -> [w2887]
    tunnel: w39 -> [w2886]
    tunnel: [w2916] -> w260
    tunnel: [w2911] -> w258
    timing: w165 -> [_]
    timing-out: [_] -> w164
    tunnel: w59 -> [w2724]
    stop <- "Stop All" stop-if-true
    w2639 = "Initialize"
    w2709 = "NI_ChannelName" ("name")
    n1689 = node-c288() -> ()  [unwired: 2 out]
    n1690 = First Call?() -> (First Call?: T/F=w2674:bool)
    n1691 = Or(x="Reset", y=w2674) -> (x .or. y?=w2675:bool)
    n1692 = case "Reset data stream" shown="True" w2675 {
      tunnel: w2887 -> [w3858 w3866]
      tunnel: w2886 -> [w3857 w3865]
      tunnel: [w3858 w3860] -> w2882
      tunnel: [w3857 w3859] -> w2881
      frame False {
      }
      frame True {
        w3863 = TRUE ("AI to FIFO")
        n1693 = local write "Overflow (data lost)"(FALSE ("Overflow (data lost)")) -> ()
        n1694 = call "reset FPGA DMA.vi"("error in"=w3865, "FPGA VI Reference In"=w3866) -> ("error out"=w3861:errorcluster, "FPGA VI Reference Out"=w3862:T19)
        n1695 = xnode "Read/Write Control"("FPGA VI Reference In"=w3862, "error in"=w3861, "AI to FIFO"=w3863, "APD to FIFO"=w3863) -> ("FPGA VI Reference Out"=w3860:T19, "error out"=w3859:errorcluster)
      }
    }
    n1696 = Or(x="Start AOD Scan", y="Trap Raster Scan") -> (x .or. y?=w2832:bool)
    n1697 = case "Start AOM raster scan" shown="True" w2832 {
      tunnel: w2882 -> [w3708 w3718]
      tunnel: w2881 -> [w3707 w3717]
      tunnel: [w3708 w3711] -> w2880
      tunnel: [w3707 w3710] -> w2879
      frame False {
      }
      frame True {
        n1698 = case shown="True" "Restart DMA? (AOD)" {
          tunnel: [w3756 w3758] -> w3712
          tunnel: [w3755 w3757] -> w3713
          tunnel: w3718 -> [w3756 w3760]
          tunnel: w3717 -> [w3755 w3759]
          frame False {
          }
          frame True {
            n1699 = local write "Overflow (data lost)"(FALSE ("Overflow (data lost)")) -> ()
            n1700 = call "reset FPGA DMA.vi"("error in"=w3759, "FPGA VI Reference In"=w3760) -> ("error out"=w3757:errorcluster, "FPGA VI Reference Out"=w3758:T19)
          }
        }
        n1701 = local write "Trap Raster Scan"(FALSE ("Trap Raster Scan")) -> ()
        n1702 = case shown="True" "Move MCL Also?" {
          tunnel: w3713 -> [w3721 w3750]
          tunnel: w3712 -> [w3722 w3751]
          tunnel: [w3720 w3754] -> w3711
          tunnel: [w3719 w3753] -> w3710
          frame False {
            w3723 = TRUE ("AI to FIFO")
            n1703 = xnode "Read/Write Control"("FPGA VI Reference In"=w3722, "error in"=w3721, "AI to FIFO"=w3723, "APD to FIFO"=w3723, "Start scan"=w3723) -> ("FPGA VI Reference Out"=w3720:T19, "error out"=w3719:errorcluster)
          }
          frame True {
            w3747 = FALSE ("1D or 2D Scan?")
            w3752 = TRUE ("AI to FIFO")
            # "Count for MCL loop"
            # "N total cycles"
            # "N steps"
            # "V_int"
            n1704 = local read "Scan Range (nm)"() -> (w3729:dbl)
            n1705 = local read "Number of F/B Scans (AOD)"() -> (w3746:u16)
            n1706 = Sign(1:w3729) -> (0:w3728:dbl)
            n1707 = Compound Arithmetic op=MULTIPLY(w3729, "MCL Step Position Ratio", "MCL/AOM Scale Tweak") -> (w3733:dbl)
            n1708 = Negate(x=w3728) -> (-x=w3725:dbl)
            n1709 = Multiply(x=w3725, y="MCL Step Increment (V_int)") -> (x*y=w3727:dbl)
            n1710 = Divide(x=w3733, y="MCL X Cal (nm/V)") -> (x/y=w3739:dbl)
            n1711 = Multiply(x=32767.0 ("y"), y=w3739) -> (x*y=w3745:dbl)
            n1712 = local read "Total Counts (ticks)"() -> (w3730:u32)
            n1713 = local read "Cycles/step (AOD)"() -> (w3741:u64)
            n1714 = local read "Scan steps (AOD)"() -> (w3742:u64)
            n1715 = Divide(x=w3745, y=10.0) -> (x/y=w3738:dbl)
            n1716 = Divide(x=w3738, y="MCL Step Increment (V_int)") -> (x/y=w3736:dbl)
            n1717 = Absolute Value(x=w3736) -> (abs(x)=w3724:dbl)
            n1718 = Compound Arithmetic op=MULTIPLY(w3742, w3741, w3730) -> (w3737:u64)
            n1719 = local write "wait to reset values"(w3752) -> ()
            n1720 = local write "MCL Scanning"(w3752) -> ()
            n1721 = Divide(x=w3737, y=w3724) -> (x/y=w3734:dbl)
            "MCL Count" <- w3734
            n1722 = xnode "Read/Write Control"("FPGA VI Reference In"=w3751, "error in"=w3750, "Scan steps (MCL)"=w3724, "Number of scans (MCL)"=w3746, "Cycles per step (MCL)"=u64 1, "Scan freq.  increment (MCL)"=w3727, "1D or 2D Scan?"=w3747, "MCL Scan Axis"=w3747, "Cont. Scan (MCL)"=w3747, "MCL count"=w3734) -> ("FPGA VI Reference Out"=w3749:T19, "error out"=w3748:errorcluster)
            n1723 = xnode "Read/Write Control"("FPGA VI Reference In"=w3749, "error in"=w3748, "AI to FIFO"=w3752, "APD to FIFO"=w3752, "Start scan"=w3752, "Start scan (MCL)"=w3752) -> ("FPGA VI Reference Out"=w3754:T19, "error out"=w3753:errorcluster)
          }
        }
        "Raster Scanning..." <- TRUE ("Scanning...")
      }
    }
    n1724 = And(x="Save scans", y=w2832) -> (x .and. y?=w2878:bool)
    n1725 = Compound Arithmetic op=OR("Start MCL Scan", "Confocal Image", "Confocal Linescan") -> (w2830:bool)
    n1726 = And(x="Save Data (MCL)", y=w2830) -> (x .and. y?=w2877:bool)
    n1727 = case "Start MCL raster scan" shown="True" w2830 {
      tunnel: w2880 -> [w3325 w3341]
      tunnel: w2879 -> [w3324 w3340]
      tunnel: [w3325 w3336] -> w2722
